vi "Channels.Inline.Read.Channel Pointer.vi"(8 "error in (no error)":errorcluster, 10 "Value in (0)":dbl, 11 "Channel Pointer":u64) -> (0 "error out":errorcluster, 2 "Value out":dbl, 3 "Channel Pointer dup":u64)   [LabVIEW 2016, in "VeriStand Data.lvlib"]
doc: "Reads the channel data specified by <B>Channel Pointer</B> into the provided <B>Value</B> scalar."
uses:
  VeriStand Data.lvlib
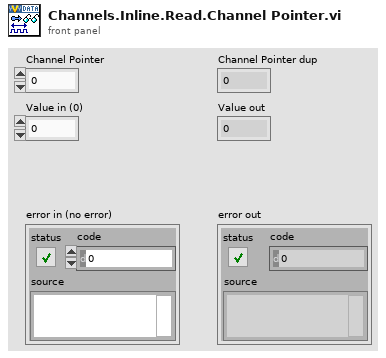
[diagram p1: front panel]
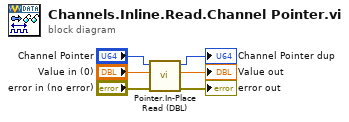
[diagram p0: block diagram]
diagram:
  n1 = call "Pointer.In-Place Read (DBL).vi"("error in (no error)"="error in (no error)", "value in"="Value in (0)", "pointer in"="Channel Pointer") -> ("error out"=→"error out":errorcluster, "value out"=→"Value out":dbl, "pointer out"=→"Channel Pointer dup":u64)  [unwired: 6 in]
